vi "Connect Websockets.vi"(6 "timeout (100ms)":i32=100, 8 "error in (no error)":errorcluster, 10 "remote port (80)":u16=80, 11 "address (localhost)":string="localhost") -> (0 "error out":errorcluster, 3 "WSConnection":refnum<class "WebsocketsConnection.lvclass">)   [LabVIEW 2013, in "MQTT_Websockets.lvlib" / "WebsocketsConnection.lvclass"]
uses:
  WebsocketsConnection.lvclass
  MQTT_Connection/Connection/Connection.lvclass
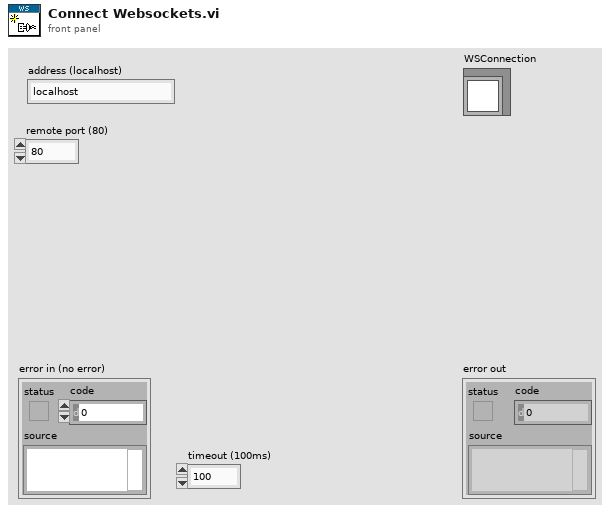
[diagram p1: front panel]
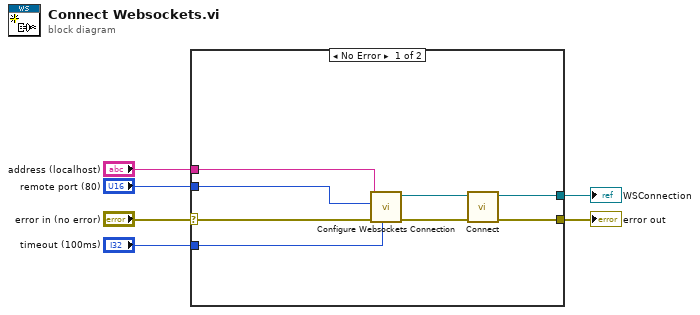
[diagram p0: block diagram]
diagram:
  n1 = case shown="No Error" "error in (no error)" {
    selector: "error in (no error)" -> [w12 w15]
    tunnel: [w13 w15] -> w5
    tunnel: [w14 _] -> w1
    tunnel: "address (localhost)" -> [w9 _]
    tunnel: "remote port (80)" -> [w8 _]
    tunnel: "timeout (100ms)" -> [w10 _]
    frame No Error {
      n2 = call "Configure Websockets Connection.vi"("timeout (1000 ms)"=w10, "error in (no error)"=w12, "remote port (80)"=w8, "address (localhost)"=w9) -> ("error out"=w11:errorcluster, "TCPConnection"=w7:refnum<class "WebsocketsConnection.lvclass">)  [unwired: 6 in]
      n3 = call "Connect.vi"("error in (no error)"=w11, "Connection in"=w7) -> ("error out"=w13:errorcluster, "Connection out"=w14:refnum<class "WebsocketsConnection.lvclass">)  [unwired: 8 in]
    }
    frame Error {
    }
  }
  "error out" <- w5
  "WSConnection" <- w1
